vi "Initialize Listener.vi"(8 "error in (no error)":errorcluster, 11 "ServerListener in":refnum<class "ServerListener.lvclass">) -> (0 "error out":errorcluster, 2 "listener ID":refnum<k5>, 3 "ServerListener out":refnum<class "ServerListener.lvclass">)   [LabVIEW 2016, in "ServerListener.lvlib" / "ServerListener.lvclass"]
uses:
  ServerListener.lvclass
  C:/Program Files (x86)/National Instruments/LabVIEW 2016/vi.lib/ActorFramework/Actor/Actor.lvclass
  ServerListener.lvclass/ServerListener.ctl
  <vilib>/ActorFramework/Actor/Actor.lvclass/Actor.ctl
  <vilib>/ActorFramework/Message Enqueuer/Message Enqueuer.lvclass/Message Enqueuer.ctl
  <vilib>/ActorFramework/Message Enqueuer/Enqueue.vi
  Controller/Messages/Listener Online Msg/Listener Online Msg.lvclass
  C:/Program Files (x86)/National Instruments/LabVIEW 2016/vi.lib/ActorFramework/Message/Message.lvclass
  <vilib>/ActorFramework/Message Priority Queue/Priority Enqueue.vi
  <vilib>/ActorFramework/Actor/Actor.lvclass
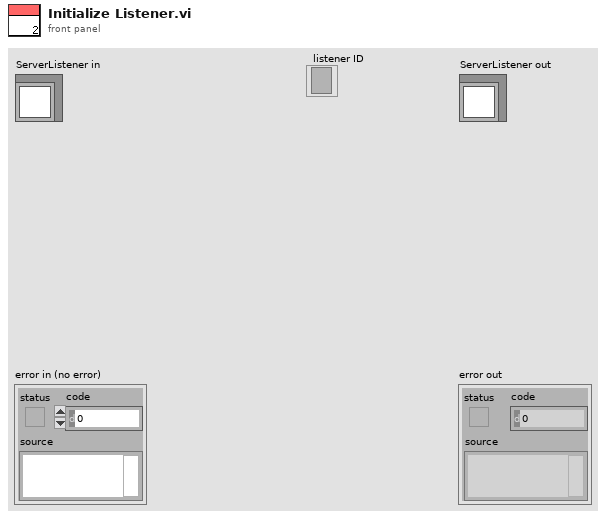
[diagram p1: front panel]
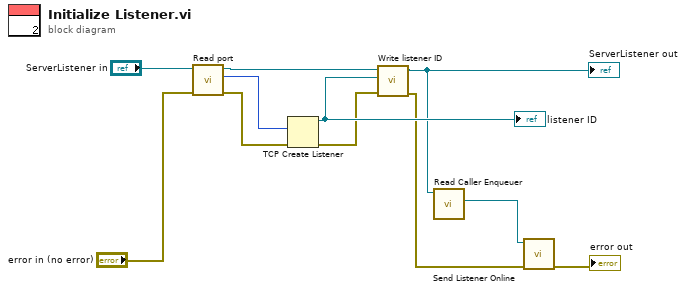
[diagram p0: block diagram]
diagram:
  n1 = call "Read port.vi"("error in (no error)"="error in (no error)", "ServerListener in"="ServerListener in") -> ("error out"=w6:errorcluster, "port"=w10:u16, "ServerListener out"=w9:refnum<class "ServerListener.lvclass">)  [unwired: 7 in]
  n2 = TCP Create Listener(8:w6, 10:w10) -> (0:w5:errorcluster, 3:w8:refnum<k5>)  [unwired: 3 in, 1 out]
  "listener ID" <- w8
  n3 = call "Write listener ID.vi"("error in (no error)"=w5, "listener ID"=w8, "ServerListener in"=w9) -> ("error out"=w1:errorcluster, "ServerListener out"=w2:refnum<class "ServerListener.lvclass">)  [unwired: 7 in]
  "ServerListener out" <- w2
  n4 = call <vilib>:"Read Caller Enqueuer.vi"("Actor"=w2) -> ("Caller Enqueuer"=w3:refnum<class "Message Enqueuer.lvclass">)  [unwired: 10 in]
  n5 = call "Send Listener Online.vi"("error in (no error)"=w1, "Message Enqueuer"=w3) -> ("error out"=→"error out":errorcluster)  [unwired: 8 in, 1 out]
